vi "Flock_Shared_Read Value.vi"(8 "error in (no error)":errorcluster, 10 "timeout (1ms)":i32=1) -> (0 "error out":errorcluster, 1 "Exit Process":bool, 2 "Message Value":string, 3 "Message Name":string)   [LabVIEW 2013, in "Flock_Shared_Messaging.lvlib" / "Flock_Shared_CentralProcessMessaging.lvlib"]
uses:
  Flock_Shared_CentralProcessMessaging.lvlib
  FGV_Action.ctl
  Flock_Shared_Messaging.lvlib
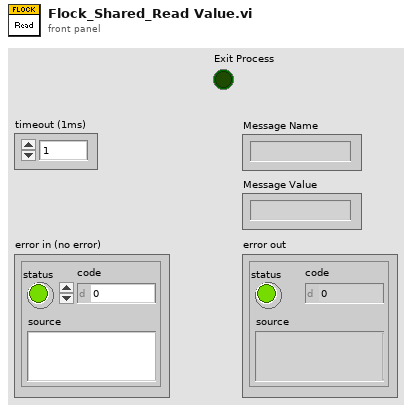
[diagram p1: front panel]
types:
  T1 = typedef "FGV_Action.ctl" = enum16{"Initalize Central", "Initialize Local", "Get", "Delete Local"}
  T2 = typedef "amc_Message Queue.ctl" = refnum<queue>
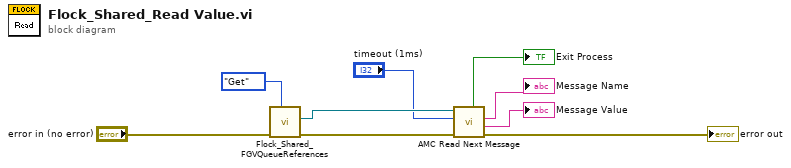
[diagram p0: block diagram]
diagram:
  n1 = call "Flock_Shared_FGVQueueReferences.vi"("Action"=FGV_Action."Get", "error in (no error)"="error in (no error)") -> ("error out"=w5:errorcluster, "Central Queue out"=w3:T2)  [unwired: 7 in, 1 out]
  n2 = call <vilib>:"AMC Read Next Message.vi"("error in (no error)"=w5, "timeout (1ms)"="timeout (1ms)", "Message Queue in"=w3) -> ("error out"=→"error out":errorcluster, "Message Value"=→"Message Value":string, "Message Name"=→"Message Name":string, "Exit Process"=→"Exit Process":bool)  [unwired: 2 in, 3 out]
